vi "CheckSubpanelDirectory.vi"(8 "error in (no error)":errorcluster, 11 "Path":path) -> (0 "error out":errorcluster, 1 "Subpanels Found?":bool, 2 "Array":path[](array[path]), 3 "Path":path)   [LabVIEW 2020, in "SMO.UI.MAUI.lvclass"]
uses:
  SMO.UI.MAUI.lvclass
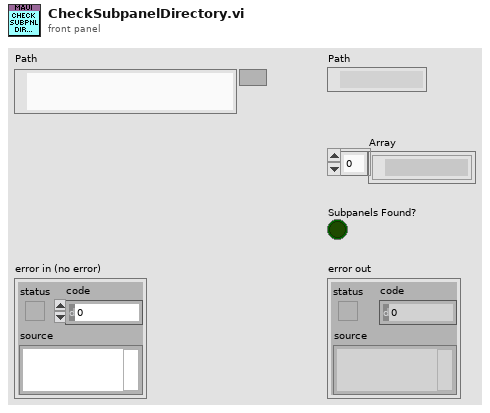
[diagram p1: front panel]
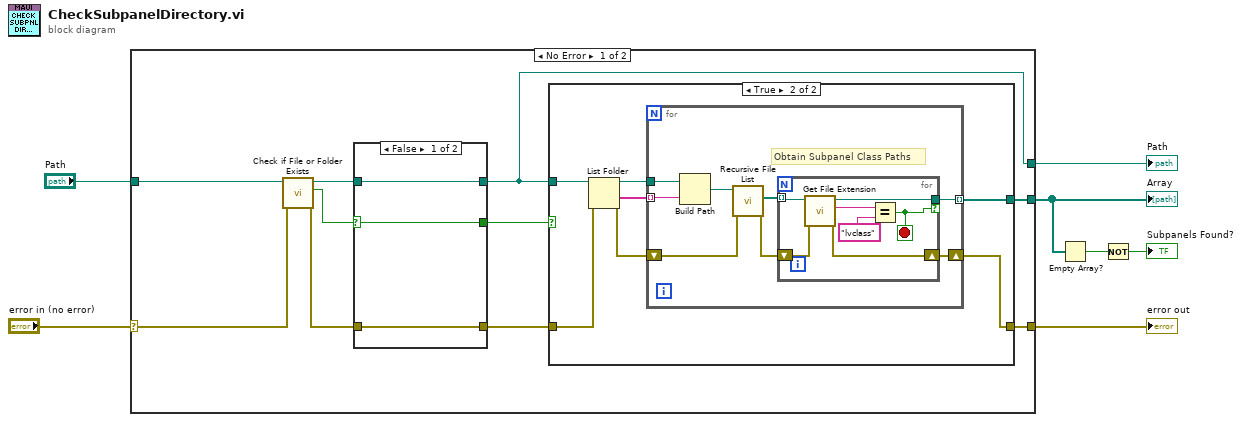
[diagram p0: block diagram]
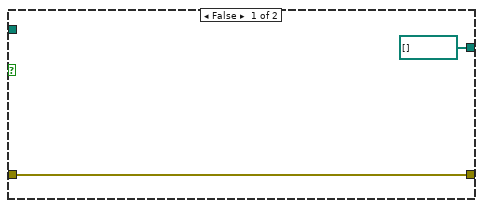
[diagram p2: hidden frame]
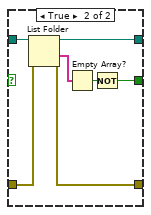
[diagram p3: hidden frame]
diagram:
  n1 = case shown="No Error" "error in (no error)" {
    selector: "error in (no error)" -> [w14 w53]
    tunnel: [w11 w53] -> w6
    tunnel: "Path" -> [w13 w52]
    tunnel: [w10 _] -> w4
    tunnel: [w8 w52] -> w3
    frame No Error {
      n2 = call <vilib>:"Check if File or Folder Exists.vi"("error in (no error)"=w14, "path"=w13) -> ("error out"=w16:errorcluster, "file or folder exists?"=w15:bool, "dup path"=w17:path)  [unwired: 7 in]
      n3 = case shown="False" w15 {
        selector: w15 -> [w43 _]
        tunnel: w17 -> [w42 w51]
        tunnel: w16 -> [w44 w50]
        tunnel: [w44 w49] -> w12
        tunnel: [w43 w47] -> w9
        tunnel: [w42 w46] -> w8
        frame False {
        }
        frame True {
          n4 = List Folder(path=w51, error in=w50) -> (path out=w46:path, folder names=w45:string[], error out=w49:errorcluster)  [unwired: 2 in, 1 out]
          n5 = Empty Array?(array=w45) -> (empty?=w48:bool)
          n6 = Not(x=w48) -> (.not. x?=w47:bool)
        }
      }
      n7 = case shown="True" w9 {
        tunnel: w8 -> [_ w26]
        tunnel: w12 -> [w19 w23]
        tunnel: [w19 w21] -> w11
        tunnel: [path[] [] w20] -> w10
        frame False {
        }
        frame True {
          n8 = List Folder(path=w26, error in=w23) -> (path out=w24:path, folder names=w25:string[], error out=w22:errorcluster)  [unwired: 2 in, 1 out]
          n9 = for {
            tunnel: w25 -> [w31] mode=indexing
            tunnel: w24 -> [w30]
            shift-right: [w29] -> w21
            shift-left: w22 -> [w28]
            tunnel: [w27] -> w20 mode=indexing
            # "Obtain Subpanel Class Paths"
            n10 = Build Path(base path=w30, name or relative path=w31) -> (appended path=w32:path)
            n11 = call <vilib>:"Recursive File List.vi"("error in (no error)"=w28, "Folder Path"=w32) -> ("error out"=w34:errorcluster, "All Files in Dir"=w33:path[])  [unwired: 5 in, 3 out]
            n12 = for {
              tunnel: w33 -> [w39] mode=indexing
              tunnel: [w38] -> w27 if=w35
              shift-right: [w36] -> w29
              shift-left: w34 -> [w37]
              stop <- w35 stop-if-true
              n13 = call <vilib>:"Get File Extension.vi"("error in (no error)"=w37, "file"=w39) -> ("error out"=w36:errorcluster, "lowercase file extension"=w41:string, "dup file"=w38:path)  [unwired: 5 in, 2 out]
              n14 = Equal?(x=w41, y="lvclass") -> (x = y?=w35:bool)
            }
          }
        }
      }
    }
    frame Error {
    }
  }
  "error out" <- w6
  "Array" <- w4
  "Path" <- w3
  n15 = Empty Array?(array=w4) -> (empty?=w2:bool)
  n16 = Not(x=w2) -> (.not. x?=→"Subpanels Found?":bool)
